vi "RTD_volts-to-temp-v2-SA-1-RTD.vi"(11 "RTD Volts":dbl) -> (3 "Temp":dbl)   [LabVIEW 2023]
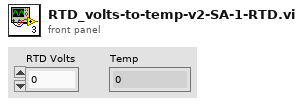
[diagram p1: front panel]
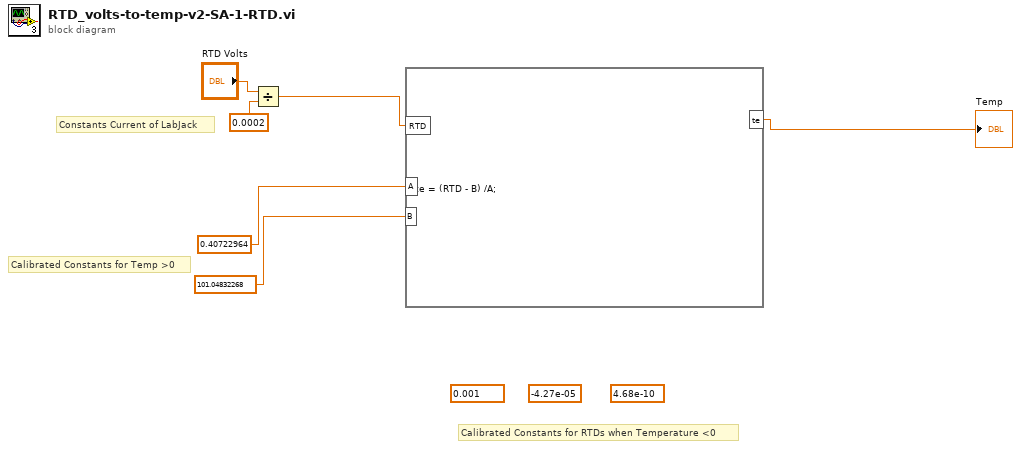
[diagram p0: block diagram]
diagram:
  (unwired) 0.001 ("y")
  (unwired) -4.27e-05 ("y")
  (unwired) 4.68e-10 ("y")
  # "Constants Current of LabJack"
  # "Calibrated Constants for Temp >0"
  # "Calibrated Constants for RTDs when Temperature <0"
  n1 = Divide(x="RTD Volts", y=0.0002) -> (x/y=w1:dbl)
  n2 = formula code="te = (RTD - B) /A;" ("DEFAULT RTD CONVERSION")("RTD"=w1, "A"=0.40722964 ("y"), "B"=101.04832268 ("y")) -> ("te"=→"Temp":dbl)
